vi "SetWavelength.vi"(0 "LambdaIn":dbl=1064.0 min=0.0 max=1000.0 step=1.0 format="%#.0f", 1 "LambdaMax":i16=25000, 2 "LambdaMin":i16=190, 3 "Sensor?":bool, 4 "RespIn":dbl=1064.0 min=1e-07 max=10000.0 step=1.0 format="%_4p", 7 "Type":u16) -> (5 "LambdaOut":dbl=10600.0 min=0.0 max=1000.0, 6 "RespOut":dbl=10600.0 min=400.0 max=1100.0)   [LabVIEW 2015]
panel:
  out "Unit":string
  out "Head":string
  in  "stop":bool
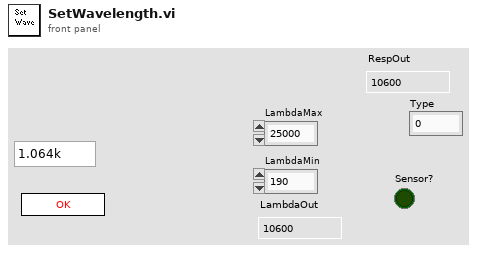
[diagram p1: front panel]
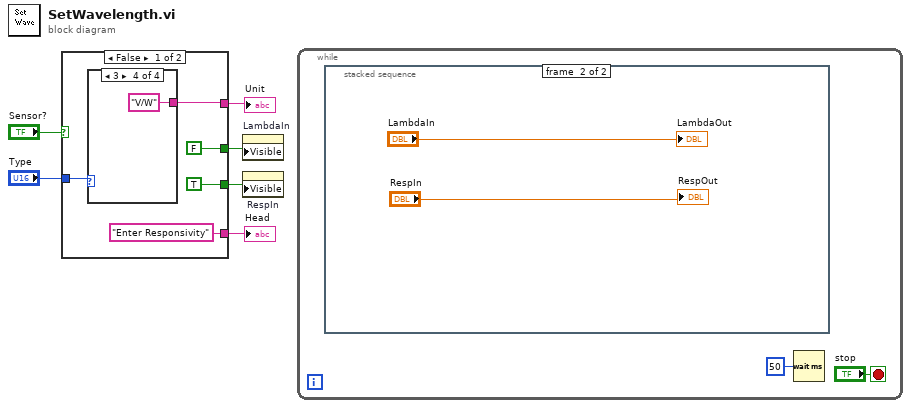
[diagram p0: block diagram]
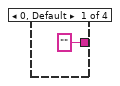
[diagram p2: hidden frame]
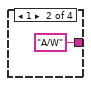
[diagram p3: hidden frame]
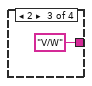
[diagram p4: hidden frame]
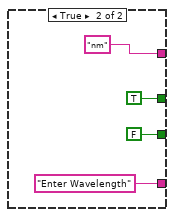
[diagram p5: hidden frame]
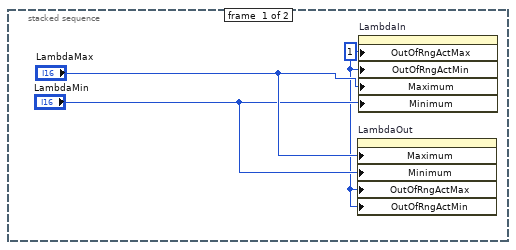
[diagram p6: hidden frame]
diagram:
  n1 = case shown="False" "Sensor?" {
    tunnel: [w7 "nm"] -> w5
    tunnel: ["Enter Responsivity" "Enter Wavelength"] -> w4
    tunnel: [TRUE FALSE] -> w3
    tunnel: [FALSE TRUE] -> w2
    tunnel: "Type" -> [w8 _]
    frame False {
      n2 = case shown="3" w8 {
        tunnel: ["" "A/W" "V/W" "V/W"] -> w7
        frame 0, Default {
        }
        frame 1 {
        }
        frame 2 {
        }
        frame 3 {
        }
      }
    }
    frame True {
    }
  }
  "Head" <- w4
  "Unit" <- w5
  n3 = property on="LambdaIn" class="DigNum (strict)"("Visible"=w2) -> ()  [unwired: 2 in, 2 out]
  n4 = property on="RespIn" class="DigNum (strict)"("Visible"=w3) -> ()  [unwired: 2 in, 2 out]
  n5 = while {
    stop <- "stop" stop-if-true
    n6 = stacked-sequence {
      frame #0 {
        w22 = u8 1 ("Response to Value Outside Limits:Maximum")
        n7 = property on="LambdaOut" class="DigNum (strict)"("Maximum"="LambdaMax", "Minimum"="LambdaMin", "OutOfRngActMax"=w22, "OutOfRngActMin"=w22) -> ()  [unwired: 2 in, 2 out]
        n8 = property on="LambdaIn" class="DigNum (strict)"("OutOfRngActMax"=w22, "OutOfRngActMin"=w22, "Maximum"="LambdaMax", "Minimum"="LambdaMin") -> ()  [unwired: 2 in, 2 out]
      }
      frame #1 {
        "LambdaOut" <- "LambdaIn"
        "RespOut" <- "RespIn"
      }
    }
    n9 = Wait (ms)(milliseconds to wait=u32 50) -> ()  [unwired: 1 out]
  }
